vi "Get MessagePrefix.vi"(8 "error in (no error)":errorcluster, 11 "PrefixQueue in":refnum<class "PrefixQueue.lvclass">) -> (0 "error out":errorcluster, 2 "MsgPrefix":string, 3 "PrefixQueue out":refnum<class "PrefixQueue.lvclass">)   [LabVIEW 2017, in "LapDog.Messaging.v3.PrefixQueue.lvlib" / "PrefixQueue.lvclass"]
uses:
  PrefixQueue.lvclass
  PrefixQueue.lvclass/PrefixQueue.ctl
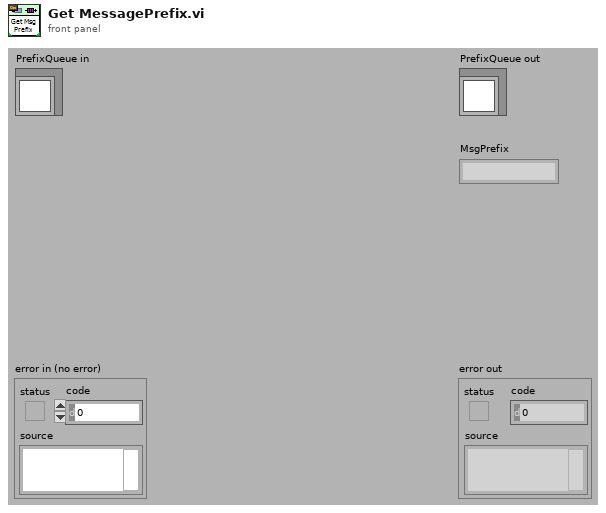
[diagram p1: front panel]
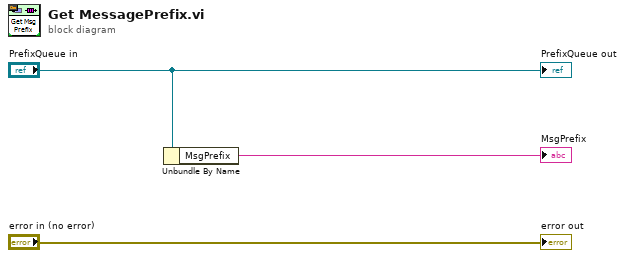
[diagram p0: block diagram]
diagram:
  n1 = Unbundle By Name("PrefixQueue in") -> ("MsgPrefix"=→"MsgPrefix":string)
  "error out" <- "error in (no error)"
  "PrefixQueue out" <- "PrefixQueue in"
